vi "KineticsCan.vi"(8 "error in":errorcluster) -> (0 "error out":errorcluster, 1 "Version":string, 3 "Res_Pass_T":bool=TRUE, 5 "Config_CANAT_out":refnum<vi>)   [LabVIEW 2017]
uses:
  PCAN_Driver/ControlCAN.llb/DevType.ctl
  PCAN_Driver/ControlCAN.llb/CAN Channel.ctl
  PCAN_Driver/ControlCAN.llb/VCI_INIT_CONFIG.ctl
  PCAN_Driver/ControlCAN.llb/InitFlag.ctl
  PCAN_Driver/ControlCAN.llb/Fliter.ctl
  PCAN_Driver/ControlCAN.llb/Mode.ctl
  PCAN_Driver/ControlCAN.lvlib
panel:
  out "Data out":u8[](array[numeric])
  out "Config_CANAT":T7 {"DevType" items=["USB-CAN"=3, "USB-CAN2"=4]; "CanIndex" items=["通道1", "通道2"]; "VCI_INIT_CONFIG"."Fliter" items=["接收所有类型"=3, "只接收标准帧"=4, "只接收扩展帧"=7]; "VCI_INIT_CONFIG"."Mode" items=["正常工作", "自测模式（环回）", "仅侦听模式"]; "VCI_INIT_CONFIG"."InitFlag" items=["使用Flash参数", "使用界面设置参数"]}
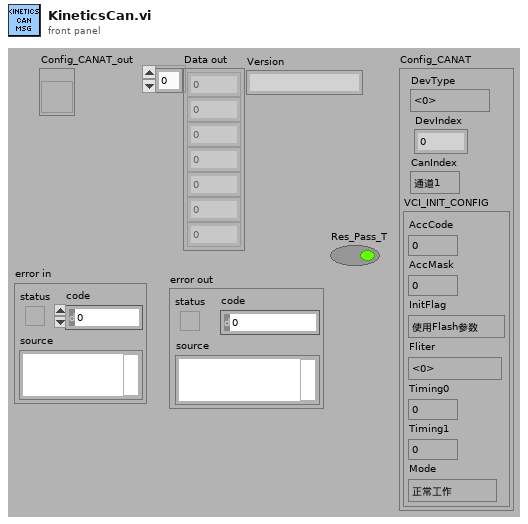
[diagram p1: front panel]
types:
  T1 = typedef "ControlCAN.lvlib/DevType.ctl" = u32
  T2 = typedef "ControlCAN.lvlib/CAN Channel.ctl" = u32
  T3 = typedef "ControlCAN.lvlib/VCI_INIT_CONFIG.ctl" = cluster{"AccCode":u32, "AccMask":u32, "InitFlag":T4, "Fliter":T5, "Timing0":u8, "Timing1":u8, "Mode":T6}
  T4 = typedef "ControlCAN.lvlib/InitFlag.ctl" = u32
  T5 = typedef "ControlCAN.lvlib/Fliter.ctl" = u8
  T6 = typedef "ControlCAN.lvlib/Mode.ctl" = u8
  T7 = cluster{"DevType":T1, "DevIndex":u32, "CanIndex":T2, "VCI_INIT_CONFIG":T3}
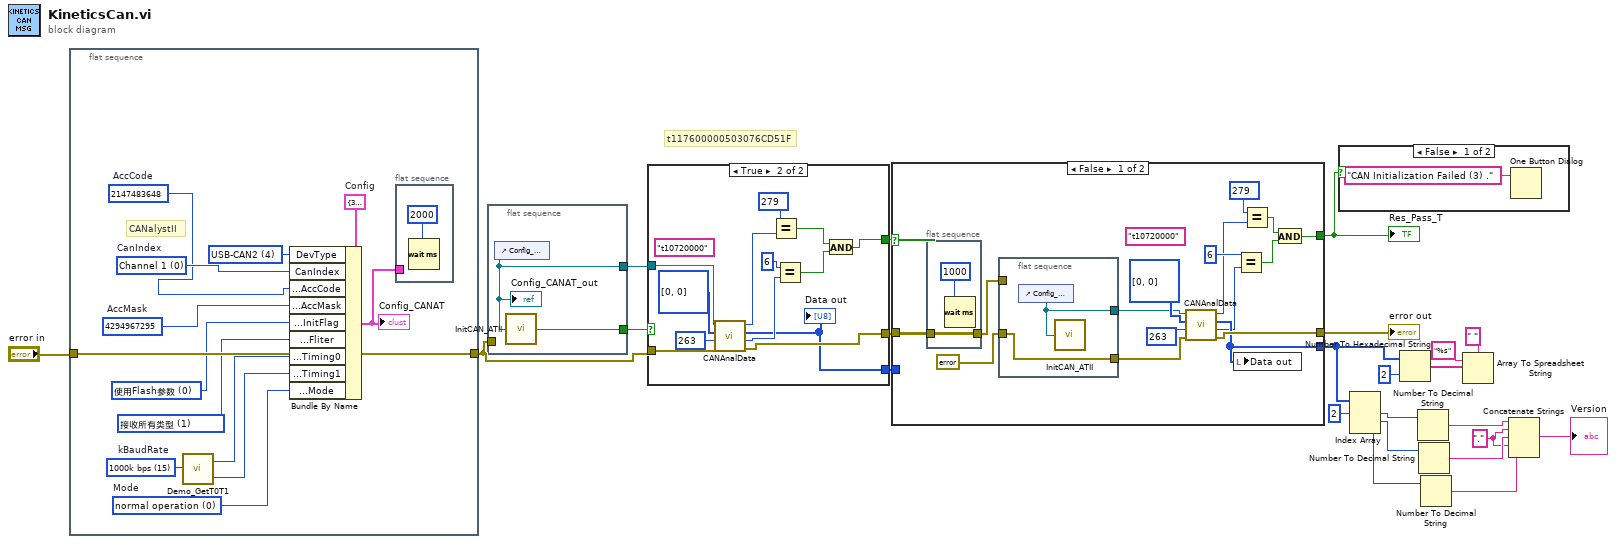
[diagram p0: block diagram]
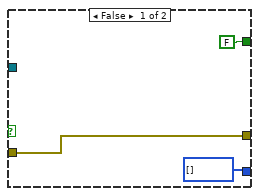
[diagram p4: hidden frame]
diagram:
  w2 = "."
  # "t117600000503076CD51F"
  n1 = flat-sequence {
    tunnel: "error in" -> [w36]
    tunnel: [w36] -> w17
    frame #0 {
      w24 = u32 2147483648  # AccCode
      w26 = T2 0 items=["Channel 1", "Channel 2"]  # CanIndex
      w29 = u32 4294967295  # AccMask
      w30 = T4 0 items=["使用Flash参数", "使用界面设置参数"] ("InitFlag")
      w35 = T6 0 items=["normal operation", "Listen-only mode", "test mode"]  # Mode
      w31 = T5 1 items=["接收所有类型"=1, "只接收标准帧"=2, "只接收扩展帧"=3] ("Fliter")
      w32 = u8 15 items=["5k bps"=1, "10k bps"=2, "20k bps"=3, "40k bps"=4, "50k bps"=5, "80k bps"=6, "100k bps"=7, "125k bps"=8, "200k bps"=9, "250k bps"=10, "400k bps"=11, "500k bps"=12, "666k bps"=13, "800k bps"=14, "1000k bps"=15, "33.33k bps"=16, "66.66k bps"=17, "83.33k bps"=18]  # kBaudRate
      w28 = T1 4 items=["USB-CAN"=3, "USB-CAN2"=4] ("DevType")
      w27 = T7 {"DevType"=3, "DevIndex"=0, "CanIndex"=0, "VCI_INIT_CONFIG"={"AccCode"=0, "AccMask"=0, "InitFlag"=1, "Fliter"=3, "Timing0"=0, "Timing1"=0, "Mode"=0}}  # Config
      # "CANalystII"
      n2 = call "Demo_GetT0T1.vi"("kBaudRate"=w32) -> ("Timing0"=w33:u8, "Timing1"=w34:u8)
      n3 = Bundle By Name(cluster=w27, "DevType"=w28, "CanIndex"=w26, "VCI_INIT_CONFIG.AccCode"=w24, "VCI_INIT_CONFIG.AccMask"=w29, "VCI_INIT_CONFIG.InitFlag"=w30, "VCI_INIT_CONFIG.Fliter"=w31, "VCI_INIT_CONFIG.Timing0"=w33, "VCI_INIT_CONFIG.Timing1"=w34, "VCI_INIT_CONFIG.Mode"=w35) -> (w25:T7)
      "Config_CANAT" <- w25
      n4 = flat-sequence {
        tunnel: w25 -> [_]
        frame #0 {
          n5 = Wait (ms)(milliseconds to wait=u32 2000) -> ()  [unwired: 1 out]
        }
      }
    }
  }
  n6 = flat-sequence {
    tunnel: [w39] -> w23
    tunnel: [w38] -> w21
    tunnel: w17 -> [_]
    frame #0 {
      n7 = control-ref of="Config_CANAT"() -> (w38:refnum<vi>)
      "Config_CANAT_out" <- w38
      n8 = call "InitCAN_ATII.vi"("Config"=w38) -> ("Sts"=w39:bool)
    }
  }
  n9 = case shown="True" w23 {
    tunnel: w17 -> [w42 w55]
    tunnel: [w42 w54] -> w19
    tunnel: [FALSE w46] -> w20
    tunnel: w21 -> [_ w53]
    tunnel: [u8[] [] ("Data out") w43] -> w18
    frame False {
    }
    frame True {
      (unwired) "t10720000" ("write buffer")
      n10 = call "CANAnalData.vi"("error in"=w55, "ID"=u32 263, "Data"=u8[] [0, 0], "Config"=w53) -> ("error out"=w54:errorcluster, "DataLen"=w44:u8, "Data out"=w43:u8[], "ID out"=w45:u32)  [unwired: 3 in, 1 out]
      "Data out" <- w43
      n11 = Equal?(x=u32 279 ("ID"), y=w45) -> (x = y?=w48:bool)
      n12 = Equal?(x=u8 6, y=w44) -> (x = y?=w47:bool)
      n13 = And(x=w48, y=w47) -> (x .and. y?=w46:bool)
    }
  }
  n14 = case shown="False" w20 {
    selector: w20 -> [_ w78]
    tunnel: [w69 w78] -> w1
    tunnel: w19 -> [w71 w77]
    tunnel: [w70 w77] -> w15
    tunnel: [w68 w76] -> w10
    tunnel: w18 -> [_ w76]
    frame False {
      (unwired) "t10720000" ("write buffer")
      n15 = flat-sequence {
        tunnel: w71 -> [w75]
        tunnel: [w75] -> w66
        frame #0 {
          n16 = Wait (ms)(milliseconds to wait=u32 1000) -> ()  [unwired: 1 out]
        }
      }
      n17 = flat-sequence {
        tunnel: errorcluster {"status"=FALSE, "code"=0, "source"=""} ("error out 4") -> [w73]
        tunnel: [w73] -> w63
        tunnel: w66 -> [_]
        tunnel: [w72] -> w61
        frame #0 {
          n18 = control-ref of="Config_CANAT"() -> (w72:refnum<vi>)
          n19 = call "InitCAN_ATII.vi"("Config"=w72) -> ()  [unwired: 1 out]
        }
      }
      n20 = call "CANAnalData.vi"("error in"=w63, "ID"=u32 263, "Data"=u8[] [0, 0], "Config"=w61) -> ("error out"=w70:errorcluster, "DataLen"=w56:u8, "Data out"=w68:u8[], "ID out"=w57:u32)  [unwired: 3 in, 1 out]
      n21 = local write "Data out"(w68) -> ()
      n22 = Equal?(x=u8 6, y=w56) -> (x = y?=w65:bool)
      n23 = Equal?(x=u32 279 ("ID"), y=w57) -> (x = y?=w59:bool)
      n24 = And(x=w59, y=w65) -> (x .and. y?=w69:bool)
    }
    frame True {
    }
  }
  "error out" <- w15
  "Res_Pass_T" <- w1
  n25 = case shown="False" w1 {
    frame False {
      n26 = One Button Dialog(message="CAN Initialization Failed (3) .") -> ()  [unwired: 1 in, 1 out]
    }
    frame True {
    }
  }
  n27 = Index Array(array=w10, index #1=2 ("index")) -> (element #1=w8:u8, element #2=w7:u8, element #3=w6:u8)  [unwired: 2 in]
  n28 = Number To Hexadecimal String(1:i16 2 ("width (-)"), 2:w10) -> (0:w13:string[])
  n29 = Number To Decimal String(number=w8) -> (decimal integer string=w5:string)  [unwired: 1 in]
  n30 = Number To Decimal String(number=w7) -> (decimal integer string=w4:string)  [unwired: 1 in]
  n31 = Number To Decimal String(number=w6) -> (decimal integer string=w3:string)  [unwired: 1 in]
  n32 = Array To Spreadsheet String(delimiter (Tab)=" ", array=w13, 3:"%s" ("format string")) -> ()  [unwired: 1 out]
  n33 = Concatenate Strings(w5, w2, w4, w2, w3) -> (→"Version":string)
